vi "System_Inj_Array_Split.vi"(10 "Inject_Arrays":dbl[](array[numeric]), 11 "Omicron":bool) -> (0 "Valve 3":dbl[](array[numeric]), 1 "Valve 2":dbl[](array[numeric]), 2 "Valve 1":dbl[](array[numeric]), 3 "HC Bal":dbl[](array[numeric]), 4 "Evac 1":dbl[](array[numeric]), 5 "Air Bal":dbl[](array[numeric]), 6 "Evac 2":dbl[](array[numeric]), 9 "Cycle Length":i32)   [LabVIEW 2014]
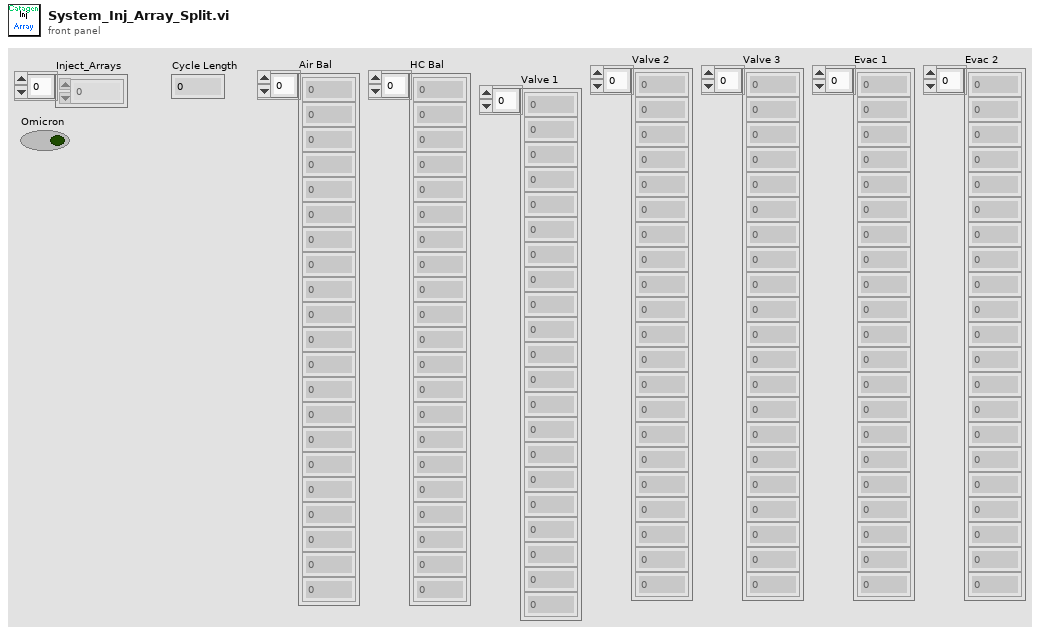
[diagram p1: front panel]
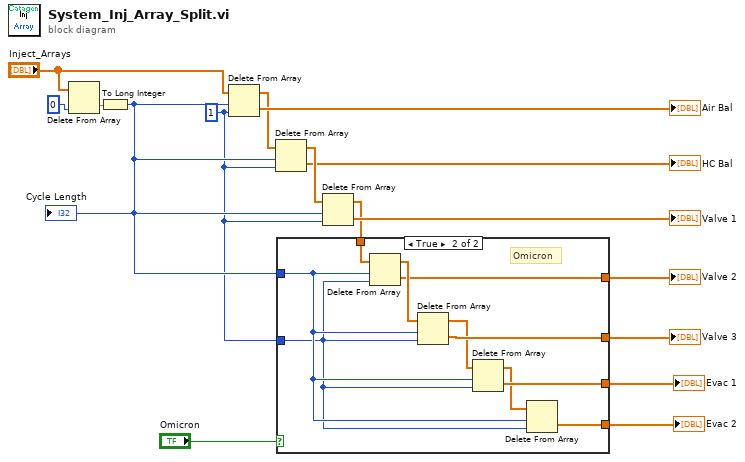
[diagram p0: block diagram]
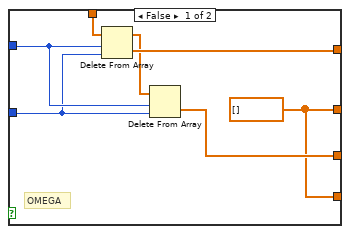
[diagram p2: hidden frame]
diagram:
  w2 = 1 ("index")
  n1 = Delete From Array(array="Inject_Arrays", index=0) -> (deleted portion=w10:dbl)  [unwired: 1 in, 1 out]
  n2 = To Long Integer(number=w10) -> (32bit integer=w3:i32)
  "Cycle Length" <- w3
  n3 = Delete From Array(array="Inject_Arrays", length=w3, index=w2) -> (deleted portion=→"Air Bal":dbl[], array with subset deleted=w15:dbl[])
  n4 = Delete From Array(array=w15, length=w3, index=w2) -> (deleted portion=→"HC Bal":dbl[], array with subset deleted=w14:dbl[])
  n5 = Delete From Array(array=w14, length=w3, index=w2) -> (deleted portion=→"Valve 1":dbl[], array with subset deleted=w11:dbl[])
  n6 = case shown="True" "Omicron" {
    tunnel: w11 -> [w23 w33]
    tunnel: [w22 w31] -> w7
    tunnel: [w17 w30] -> w6
    tunnel: [w20 w29] -> w5
    tunnel: [w17 w27] -> w4
    tunnel: w3 -> [w19 w25]
    tunnel: w2 -> [w18 w24]
    frame False {
      w17 = dbl[] [] ("Inject_Arrays")
      # "OMEGA"
      n7 = Delete From Array(array=w23, length=w19, index=w18) -> (deleted portion=w22:dbl[], array with subset deleted=w21:dbl[])
      n8 = Delete From Array(array=w21, length=w19, index=w18) -> (deleted portion=w20:dbl[])  [unwired: 1 out]
    }
    frame True {
      # "Omicron"
      n9 = Delete From Array(array=w33, length=w25, index=w24) -> (deleted portion=w31:dbl[], array with subset deleted=w32:dbl[])
      n10 = Delete From Array(array=w32, length=w25, index=w24) -> (deleted portion=w30:dbl[], array with subset deleted=w28:dbl[])
      n11 = Delete From Array(array=w28, length=w25, index=w24) -> (deleted portion=w29:dbl[], array with subset deleted=w26:dbl[])
      n12 = Delete From Array(array=w26, length=w25, index=w24) -> (deleted portion=w27:dbl[])  [unwired: 1 out]
    }
  }
  "Valve 2" <- w7
  "Valve 3" <- w6
  "Evac 1" <- w5
  "Evac 2" <- w4
